vi "REFs Name to ref convert.vi"(11 "Array in":string[](array[string])) -> (3 "Array out":refnum<vi>[](array[refnum]))   [LabVIEW 2020]
uses:
  PCT FGV CMD.ctl
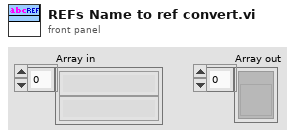
[diagram p1: front panel]
types:
  T1 = typedef "PCT FGV CMD.ctl" = enum16{"INIT", "GET", "SET"}
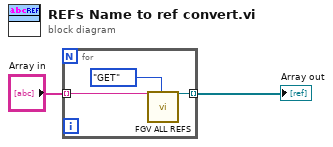
[diagram p0: block diagram]
diagram:
  n1 = for {
    tunnel: "Array in" -> [w4] mode=indexing
    tunnel: [w3] -> w1 mode=indexing
    n2 = call "FGV ALL REFS.vi"("name"=w4, "CMD"=PCT_FGV_CMD."GET") -> ("Ctl Refnum out"=w3:refnum<vi>)  [unwired: 25 in]
  }
  "Array out" <- w1
